vi "AB_RW_Convert_Path_to_Absolute.vi"(8 "error in (no error)":errorcluster, 9 "relativeType":string, 10 "commonPath":path, 11 "relativePath":path) -> (0 "error out":errorcluster, 3 "absolute path":path)   [LabVIEW 2020]
uses:
  <vilib>/AppBuilder/AB_Relative_Path_Type.ctl
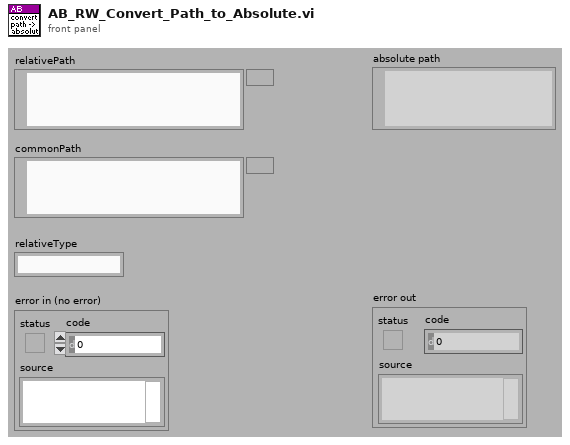
[diagram p1: front panel]
types:
  T1 = typedef "AB_Relative_Path_Type.ctl" = enum16{"<none>", "relativeToCommon", "relativeToAppDir", "relativeToProject"}
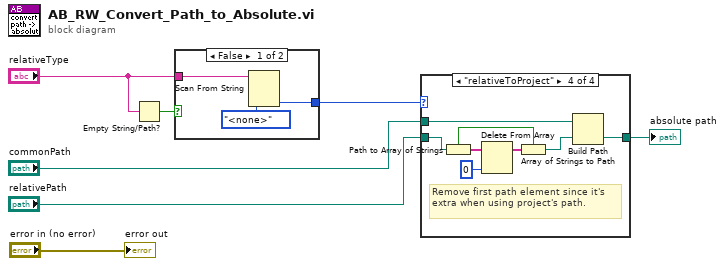
[diagram p0: block diagram]
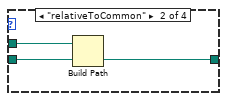
[diagram p3: hidden frame]
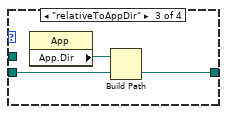
[diagram p4: hidden frame]
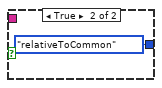
[diagram p5: hidden frame]
diagram:
  n1 = Empty String/Path?(string/path="relativeType") -> (empty?=w2:bool)
  n2 = case shown="False" w2 {
    tunnel: "relativeType" -> [w9 _]
    tunnel: [w8 AB_Relative_Path_Type."relativeToCommon" ("relativeType")] -> w4
    frame False {
      n3 = Scan From String(input string=w9, default 1=AB_Relative_Path_Type."<none>" ("relativeType")) -> (output 1=w8:T1)  [unwired: 3 in, 3 out]
    }
    frame True {
    }
  }
  n4 = case shown="\"relativeToProject\"" w4 {
    tunnel: "relativePath" -> [w12 w15 w18 w20]
    tunnel: [w12 w14 w17 w26] -> w6
    tunnel: "commonPath" -> [_ w13 _ w25]
    frame "<none>" {
      # "absolute path"
    }
    frame "relativeToCommon" {
      n5 = Build Path(base path=w13, name or relative path=w15) -> (appended path=w14:path)
    }
    frame "relativeToAppDir" {
      n6 = property class="App"() -> ("App.Dir"=w16:path)  [unwired: 2 in, 2 out]
      n7 = Build Path(base path=w16, name or relative path=w18) -> (appended path=w17:path)
    }
    frame "relativeToProject" {
      # "Remove first path element since it's extra when using project's path."
      n8 = Path to Array of Strings(0:w20) -> (1:w22:bool, 2:w24:string[])
      n9 = Delete From Array(array=w24, index=0) -> (array with subset deleted=w23:string[])  [unwired: 1 in, 1 out]
      n10 = Array of Strings to Path(0:w23, 1:w22) -> (2:w19:path)
      n11 = Build Path(base path=w25, name or relative path=w19) -> (appended path=w26:path)
    }
  }
  "absolute path" <- w6
  "error out" <- "error in (no error)"
